vi "4Pi SFC - Rotate XY 45.vi"(0 "XY Amounts":dbl[](array[numeric]), 7 "Flip XY":bool, 9 "Invert X":bool, 11 "Invert Y":bool) -> (4 "45° Rotated XY":dbl[](array[numeric]))   [LabVIEW 2016]
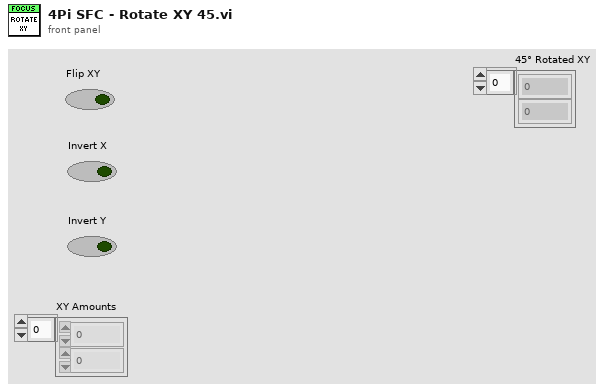
[diagram p1: front panel]
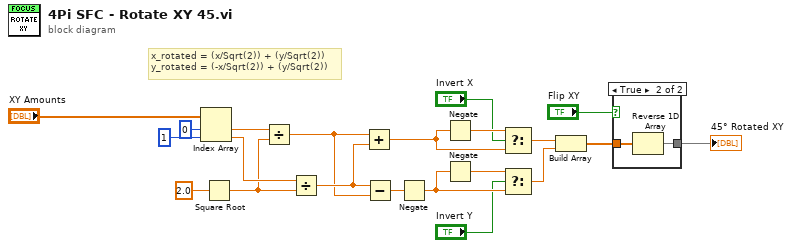
[diagram p0: block diagram]
diagram:
  # "x_rotated = (x/Sqrt(2)) + (y/Sqrt(2))\ny_rotated = (-x/Sqrt(2)) + (y/Sqrt(2))"
  n1 = Index Array(array="XY Amounts", index #1=0 ("index"), index #2=1 ("index")) -> (element #1=w19:dbl, element #2=w17:dbl)
  n2 = Square Root(x=2.0) -> (sqrt(x)=w16:dbl)
  n3 = Divide(x=w19, y=w16) -> (x/y=w14:dbl)
  n4 = Divide(x=w17, y=w16) -> (x/y=w15:dbl)
  n5 = Add(x=w14, y=w15) -> (x+y=w9:dbl)
  n6 = Subtract(x=w15, y=w14) -> (x-y=w13:dbl)
  n7 = Negate(x=w13) -> (-x=w6:dbl)
  n8 = Negate(x=w9) -> (-x=w8:dbl)
  n9 = Negate(x=w6) -> (-x=w7:dbl)
  n10 = Select(t=w8, s="Invert X", f=w9) -> (s? t:f=w11:dbl)
  n11 = Select(t=w7, s="Invert Y", f=w6) -> (s? t:f=w10:dbl)
  n12 = Build Array(w11, w10) -> (w12:dbl[])
  n13 = case shown="True" "Flip XY" {
    tunnel: w12 -> [w22 w24]
    tunnel: [w22 w23] -> w3
    frame False {
    }
    frame True {
      n14 = Reverse 1D Array(array=w24) -> (reversed array=w23:dbl[])
    }
  }
  "45° Rotated XY" <- w3
